vi "FTW-JSON-Object-DeleteAllElements.vi"(0 "JSON":T1, 11 "error in":errorcluster) -> (4 "JSON out":T1, 15 "error out":errorcluster)   [LabVIEW 2015]
uses:
  core/type/FTW-Type-JSON.ctl
panel:
  # "Inputs"
  # "Outputs"
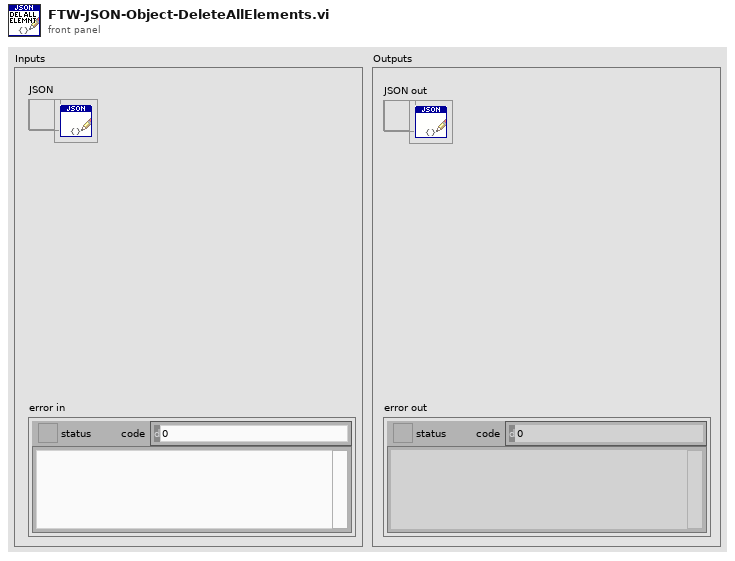
[diagram p1: front panel]
types:
  T1 = typedef "FTW-Type-JSON.ctl" = refnum<data-value>
  T2 = cluster{"FTW-CodeGen-Type":enum16{"FTW-JSON"}, "Object":i64, "EncodingFlags":i64, "DecodingFlags":i64}
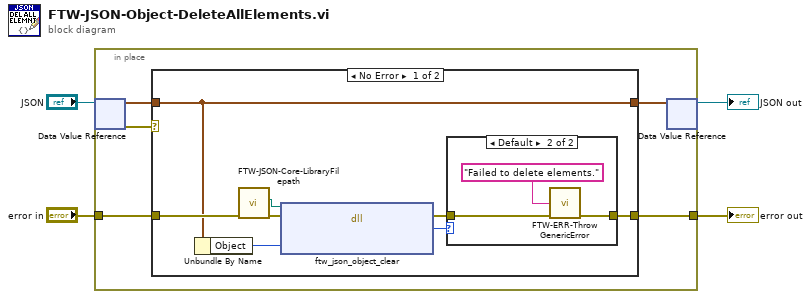
[diagram p0: block diagram]
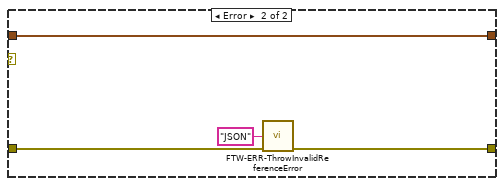
[diagram p3: hidden frame]
diagram:
  n1 = in-place {
    in-place-border: "error in" -> [w7]
    in-place-border: [w8] -> w4
    n2 = in-place-dvr #1("JSON") -> (w9:T2, w6:errorcluster)
    n3 = case shown="No Error" w6 {
      tunnel: w9 -> [w10 w22]
      tunnel: [w14 w23] -> w8
      tunnel: w7 -> [w13 w24]
      tunnel: [w10 w22] -> w5
      frame No Error {
        n4 = Unbundle By Name(w10) -> ("Object"=w17:i64)
        n5 = call "FTW-JSON-Core-LibraryFilepath.vi"("error in"=w13) -> ("error out"=w12:errorcluster, "JSON Library Filepath"=w11:path)  [unwired: 9 in]
        n6 = dll-call lib="?" fn="ftw_json_object_clear"(path in=w11, error in=w12, "JSON Object Pointer"=w17) -> (error out=w15:errorcluster, "Return Value"=w16:i64)  [unwired: 2 in, 1 out]
        n7 = case shown="Default" w16 {
          tunnel: w15 -> [w18 w21]
          tunnel: [w18 w20] -> w14
          frame 0 {
          }
          frame Default {
            n8 = call "FTW-ERR-ThrowGenericError.vi"("Error Message"="Failed to delete elements.", "error in"=w21) -> ("error out"=w20:errorcluster)  [unwired: 13 in]
          }
        }
      }
      frame Error {
        n9 = call "FTW-ERR-ThrowInvalidReferenceError.vi"("Reference Type"="JSON", "error in"=w24) -> ("error out"=w23:errorcluster)  [unwired: 13 in]
      }
    }
    n10 = in-place-dvr #1(w5) -> (→"JSON out":T1)  [unwired: 1 out]
  }
  "error out" <- w4
